vi "Send Outputs.vi"(8 "error in":errorcluster, 11 "PIOD in":refnum<class "PIOD.lvclass">) -> (0 "error out":errorcluster, 3 "PIOD out":refnum<class "PIOD.lvclass">)   [LabVIEW 2018, in "PIOD.lvlib" / "PIOD.lvclass"]
uses:
  PIOD.lvclass
  Custom Controls/File Number.ctl
  <vilib>/ethernetip/ethernetip.llb/EthernetIPSLC500FileType.ctl
  PIOD.lvclass/PIOD.ctl
  Accessors/Read/Read Timeout (ms).vi
  <vilib>/ethernetip/ethernetip.llb/EthernetIP SLC500 Write Raw.vi
  <vilib>/ethernetip/ethernetip.lvlib
  PPLs/PLC/Parent/PLC.lvlibp/PLC.lvclass
  C:/AME Test Engineering/LabVIEW/PPLs/PLC/Parent/PLC.lvlibp/PLC.lvclass
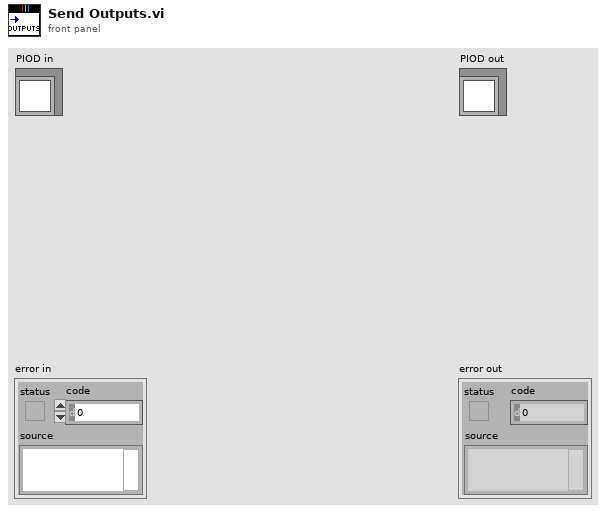
[diagram p1: front panel]
types:
  T1 = typedef "PIOD.lvlib/PIOD.lvclass/File Number.ctl" = enum16{"Output", "Input", "Status", "Output2"}
  T2 = typedef "ethernetip.lvlib/EthernetIPSLC500FileType.ctl" = u8
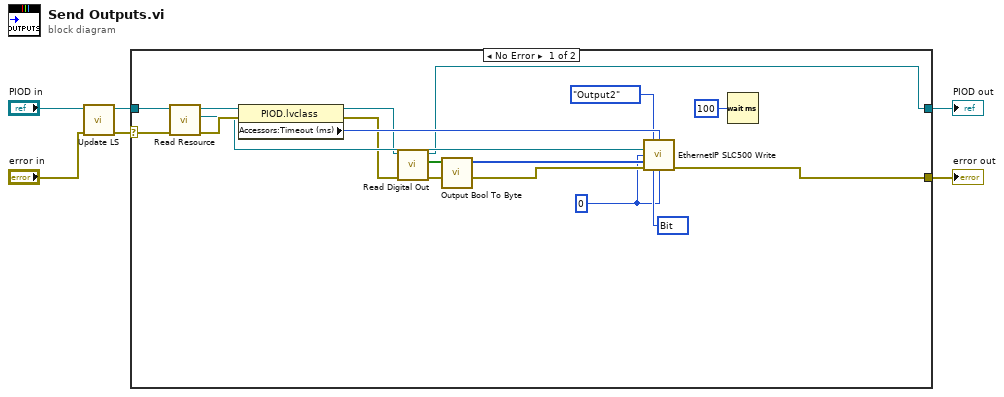
[diagram p0: block diagram]
diagram:
  n1 = call "Update LS.vi"("error in"="error in", "PIOD in"="PIOD in") -> ("error out"=w1:errorcluster, "PIOD out"=w3:refnum<class "PIOD.lvclass">)  [unwired: 8 in]
  n2 = case shown="No Error" w1 {
    selector: w1 -> [w17 w25]
    tunnel: [w23 w25] -> w6
    tunnel: [w11 w24] -> w5
    tunnel: w3 -> [w19 w24]
    frame No Error {
      w9 = T2 133 items=["Status"=132, "Bit"=133, "Timer"=134, "Counter"=135, "Control"=136, "Integer"=137, "Float"=138, "Output"=139, "Input"=140, "String"=141, "ASCII"=142] ("File Type")
      w7 = u16 0 ("Element Number")
      n3 = call "Read Resource.vi"("error in (no error)"=w17, "PLC in"=w19) -> ("error out"=w16:errorcluster, "Resource"=w15:refnum<visa-resource-name>, "PLC out"=w18:refnum<class "PIOD.lvclass">)  [unwired: 7 in]
      n4 = property class="PIOD.lvclass"(reference=w18, error in=w16) -> (reference out=w14:refnum<class "PIOD.lvclass">, error out=w12:errorcluster, "Accessors:Timeout (ms)"=w21:i32)
      n5 = call "Read Digital Out.vi"("error in"=w12, "PLC in"=w14) -> ("error out"=w13:errorcluster, "Digital Out"=w20:bool[], "PLC out"=w11:refnum<class "PIOD.lvclass">)  [unwired: 7 in]
      n6 = call "Output Bool To Byte.vi"("Output Settings"=w20) -> ("Output Settings out"=w22:u8[])  [unwired: 10 in]
      n7 = call-poly <vilib>:"EthernetIP SLC500 Write.vi"("File Number"=File_Number."Output2", "Timeout (ms)"=w21, "Network Path"=w15, "Element Number"=w7, "Data"=w22, "error in"=w13, "File Type"=w9, "Subelement Number"=w7) -> ("error out"=w23:errorcluster)  [unwired: 6 in, 1 out]
      n8 = Wait (ms)(milliseconds to wait=u32 100) -> ()  [unwired: 1 out]
    }
    frame Error {
    }
  }
  "error out" <- w6
  "PIOD out" <- w5
